vi "initialize.vi"(0 "HGF_TimeoutWorker":refnum<class "HGF_TimeoutWorker.lvclass">, 3 "initializationData":variant, 5 "error in (no error)":errorcluster, 7 "binaryString":string, 8 "I8 Array":i8[](array[numeric]), 9 "prependSize? (T)":bool, 11 "byteOrder (0:big-endian, network order)":T1(ring)) -> (14 "dup HGF_TimeoutWorker":refnum<class "HGF_TimeoutWorker.lvclass">, 17 "found?":bool, 19 "error out":errorcluster)   [LabVIEW 2014, in "HGF_BaseClasses.lvlib" / "HGF_TimeoutWorker.lvclass"]
doc: "This is a dynamic dispatch VI to be implemented by child classes to initialize their attributes.\n\n<B>Recommendation:</B> Use Variant for initialization data."
uses:
  HGF_TimeoutWorker.lvclass
  HGF_BaseClasses/HGF_ThreadWorker/HGF_ThreadWorker.lvclass
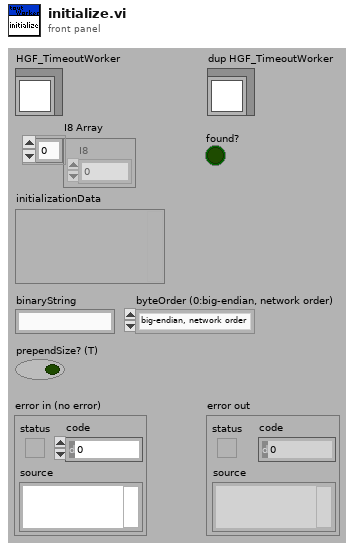
[diagram p1: front panel]
types:
  T1 = enum16{"big-endian, network order", "native, host order", "little-endian"}
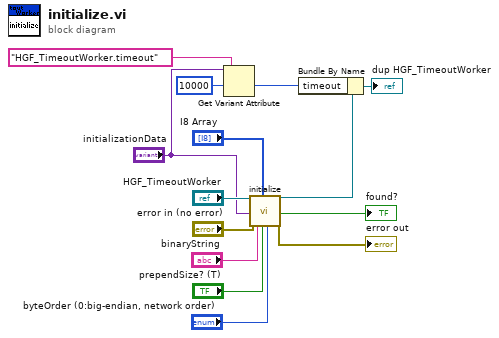
[diagram p0: block diagram]
diagram:
  n1 = Get Variant Attribute(Variant="initializationData", name="HGF_TimeoutWorker.timeout", default value (empty Variant)=10000) -> (value=w1:i32)  [unwired: 1 in, 3 out]
  n2 = call-parent "initialize.vi"("HGF_Base"="HGF_TimeoutWorker", "initializationData"="initializationData", "error in (no error)"="error in (no error)", "binaryString"="binaryString", "I8 Array"="I8 Array", "prependSize? (T)"="prependSize? (T)", "byteOrder (0:big-endian, network order)"="byteOrder (0:big-endian, network order)") -> ("dup HGF_Base"=w8:refnum<class "HGF_TimeoutWorker.lvclass">, "found?"=→"found?":bool, "error out"=→"error out":errorcluster)  [unwired: 10 in]
  n3 = Bundle By Name(cluster=w8, "timeout"=w1) -> (→"dup HGF_TimeoutWorker":refnum<class "HGF_TimeoutWorker.lvclass">)
